vi "HFRR ADV v01.vi"() -> ()   [LabVIEW 2025] (continued)
        n1012 = property on="Analysis" class="Bool (strict)"("DisabledEnum"=w970) -> ()  [unwired: 2 in, 2 out]
        n1013 = property on="Home" class="Bool (strict)"("DisabledEnum"=w970) -> ()  [unwired: 2 in, 2 out]
        n1014 = property on="Report" class="Bool (strict)"("DisabledEnum"=w970) -> ()  [unwired: 2 in, 2 out]
        n1015 = property on="Main Dashboard Buttons" class="RadioBtnsControl (strict)"("DisabledEnum"=w970) -> ()  [unwired: 2 in, 2 out]
        n1016 = case shown="True" w969 {
          tunnel: [T15."Disabled" ("Disabled") T15."Enabled" ("Disabled")] -> w968
          frame False {
          }
          frame True {
          }
        }
        n1017 = property on="About" class="Bool (strict)"("DisabledEnum"=w968) -> ()  [unwired: 2 in, 2 out]
      }
      frame "Test Setup" {
        w975 = T15."Enabled" ("Disabled")
        n1018 = local read "Service Password enable"() -> (w974:bool)
        n1019 = property on="Dashboard" class="Bool (strict)"("DisabledEnum"=T15."Disabled" ("Disabled")) -> ()  [unwired: 2 in, 2 out]
        n1020 = property on="Imaging" class="Bool (strict)"("DisabledEnum"=w975) -> ()  [unwired: 2 in, 2 out]
        n1021 = property on="Analysis" class="Bool (strict)"("DisabledEnum"=w975) -> ()  [unwired: 2 in, 2 out]
        n1022 = property on="Home" class="Bool (strict)"("DisabledEnum"=w975) -> ()  [unwired: 2 in, 2 out]
        n1023 = property on="Report" class="Bool (strict)"("DisabledEnum"=w975) -> ()  [unwired: 2 in, 2 out]
        n1024 = property on="Test Setup" class="Bool (strict)"("DisabledEnum"=w975) -> ()  [unwired: 2 in, 2 out]
        n1025 = case shown="True" w974 {
          tunnel: [T15."Disabled" ("Disabled") T15."Enabled" ("Disabled")] -> w973
          frame False {
          }
          frame True {
          }
        }
        n1026 = property on="About" class="Bool (strict)"("DisabledEnum"=w973) -> ()  [unwired: 2 in, 2 out]
      }
      frame "Adv Scar" {
        w982 = T15."Enabled" ("Disabled")
        n1027 = property on="Dashboard" class="Bool (strict)"("DisabledEnum"=T15."Disabled" ("Disabled")) -> ()  [unwired: 2 in, 2 out]
        n1028 = property on="Imaging" class="Bool (strict)"("DisabledEnum"=w982) -> ()  [unwired: 2 in, 2 out]
        n1029 = property on="Analysis" class="Bool (strict)"("DisabledEnum"=w982) -> ()  [unwired: 2 in, 2 out]
        n1030 = property on="Home" class="Bool (strict)"("DisabledEnum"=w982) -> ()  [unwired: 2 in, 2 out]
        n1031 = property on="Report" class="Bool (strict)"("DisabledEnum"=w982) -> ()  [unwired: 2 in, 2 out]
        n1032 = property on="Test Setup" class="Bool (strict)"("DisabledEnum"=w982) -> ()  [unwired: 2 in, 2 out]
        n1033 = local read "Service Password enable"() -> (w980:bool)
        n1034 = case shown="True" w980 {
          tunnel: [T15."Disabled" ("Disabled") T15."Enabled" ("Disabled")] -> w979
          frame False {
          }
          frame True {
          }
        }
        n1035 = property on="About" class="Bool (strict)"("DisabledEnum"=w979) -> ()  [unwired: 2 in, 2 out]
      }
      frame "Adv Scar Report" {
        w987 = T15."Enabled" ("Disabled")
        n1036 = property on="Dashboard" class="Bool (strict)"("DisabledEnum"=T15."Disabled" ("Disabled")) -> ()  [unwired: 2 in, 2 out]
        n1037 = property on="Imaging" class="Bool (strict)"("DisabledEnum"=w987) -> ()  [unwired: 2 in, 2 out]
        n1038 = property on="Analysis" class="Bool (strict)"("DisabledEnum"=w987) -> ()  [unwired: 2 in, 2 out]
        n1039 = property on="Home" class="Bool (strict)"("DisabledEnum"=w987) -> ()  [unwired: 2 in, 2 out]
        n1040 = property on="Report" class="Bool (strict)"("DisabledEnum"=w987) -> ()  [unwired: 2 in, 2 out]
        n1041 = property on="Test Setup" class="Bool (strict)"("DisabledEnum"=w987) -> ()  [unwired: 2 in, 2 out]
        n1042 = local read "Service Password enable"() -> (w986:bool)
        n1043 = case shown="True" w986 {
          tunnel: [T15."Disabled" ("Disabled") T15."Enabled" ("Disabled")] -> w985
          frame False {
          }
          frame True {
          }
        }
        n1044 = property on="About" class="Bool (strict)"("DisabledEnum"=w985) -> ()  [unwired: 2 in, 2 out]
      }
      frame "Compare Files" {
        w993 = T15."Enabled" ("Disabled")
        n1045 = local read "Service Password enable"() -> (w992:bool)
        n1046 = property on="Dashboard" class="Bool (strict)"("DisabledEnum"=T15."Disabled" ("Disabled")) -> ()  [unwired: 2 in, 2 out]
        n1047 = property on="Imaging" class="Bool (strict)"("DisabledEnum"=w993) -> ()  [unwired: 2 in, 2 out]
        n1048 = property on="Analysis" class="Bool (strict)"("DisabledEnum"=w993) -> ()  [unwired: 2 in, 2 out]
        n1049 = property on="Home" class="Bool (strict)"("DisabledEnum"=w993) -> ()  [unwired: 2 in, 2 out]
        n1050 = property on="Report" class="Bool (strict)"("DisabledEnum"=w993) -> ()  [unwired: 2 in, 2 out]
        n1051 = property on="Test Setup" class="Bool (strict)"("DisabledEnum"=w993) -> ()  [unwired: 2 in, 2 out]
        n1052 = case shown="True" w992 {
          tunnel: [T15."Disabled" ("Disabled") T15."Enabled" ("Disabled")] -> w991
          frame False {
          }
          frame True {
          }
        }
        n1053 = property on="About" class="Bool (strict)"("DisabledEnum"=w991) -> ()  [unwired: 2 in, 2 out]
      }
      frame "Acquire" {
        n1054 = local read "Service Password enable"() -> (w997:bool)
        n1055 = property on="Test Setup" class="Bool (strict)"("DisabledEnum"=T15."Disabled" ("Disabled")) -> ()  [unwired: 2 in, 2 out]
        n1056 = local read "Auto Start Test"() -> (w999:bool)
        n1057 = local read "RUN"() -> (w1001:bool)
        n1058 = case shown="True" w997 {
          tunnel: [T15."Disabled" ("Disabled") T15."Enabled" ("Disabled")] -> w998
          frame False {
          }
          frame True {
          }
        }
        n1059 = Or(x=w1001, y=w999) -> (x .or. y?=w1000:bool)
        n1060 = case shown="True" w1000 {
          tunnel: [T15."Enabled" ("Disabled") T15."Disabled" ("Disabled")] -> w1003
          frame False {
          }
          frame True {
          }
        }
        n1061 = property on="About" class="Bool (strict)"("DisabledEnum"=w998) -> ()  [unwired: 2 in, 2 out]
        n1062 = property on="Imaging" class="Bool (strict)"("DisabledEnum"=w1003) -> ()  [unwired: 2 in, 2 out]
        n1063 = property on="Dashboard" class="Bool (strict)"("DisabledEnum"=w1003) -> ()  [unwired: 2 in, 2 out]
        n1064 = property on="Analysis" class="Bool (strict)"("DisabledEnum"=w1003) -> ()  [unwired: 2 in, 2 out]
        n1065 = property on="Home" class="Bool (strict)"("DisabledEnum"=w1003) -> ()  [unwired: 2 in, 2 out]
        n1066 = property on="Report" class="Bool (strict)"("DisabledEnum"=w1003) -> ()  [unwired: 2 in, 2 out]
      }
      frame "About" {
        n1067 = local read "FILE"() -> (w1016:string)
        n1068 = local read "TEST FILE NAM,E SAVED"() -> (w1009:bool)
        n1069 = call <vilib>:"Trim Whitespace.vi"("string"=w1016) -> ("trimmed string"=w1015:string)  [unwired: 1 in]
        n1070 = local read "Auto Start Test"() -> (w1019:bool)
        n1071 = String Length(string=w1015) -> (length=w1014:i32)
        n1072 = Greater?(x=w1014, y=1) -> (0:w1011:bool)
        n1073 = And(x=w1011, y=w1009) -> (x .and. y?=w1010:bool)
        n1074 = local read "RUN"() -> (w1021:bool)
        n1075 = case shown="True" w1010 {
          tunnel: [T15."Disabled" ("Disabled") T15."Enabled" ("Disabled")] -> w1012
          frame False {
          }
          frame True {
          }
        }
        n1076 = Or(x=w1021, y=w1019) -> (x .or. y?=w1020:bool)
        n1077 = property on="About" class="Bool (strict)"("DisabledEnum"=T15."Enabled" ("Disabled")) -> ()  [unwired: 2 in, 2 out]
        n1078 = case shown="False" w1020 {
          tunnel: [T15."Enabled" ("Disabled") T15."Disabled" ("Disabled")] -> w1018
          frame False {
          }
          frame True {
          }
        }
        n1079 = property on="Dashboard" class="Bool (strict)"("DisabledEnum"=w1012) -> ()  [unwired: 2 in, 2 out]
        n1080 = property on="Test Setup" class="Bool (strict)"("DisabledEnum"=T15."Disabled" ("Disabled")) -> ()  [unwired: 2 in, 2 out]
        n1081 = property on="Imaging" class="Bool (strict)"("DisabledEnum"=w1018) -> ()  [unwired: 2 in, 2 out]
        n1082 = property on="Analysis" class="Bool (strict)"("DisabledEnum"=w1018) -> ()  [unwired: 2 in, 2 out]
        n1083 = property on="Home" class="Bool (strict)"("DisabledEnum"=w1018) -> ()  [unwired: 2 in, 2 out]
        n1084 = property on="Report" class="Bool (strict)"("DisabledEnum"=w1018) -> ()  [unwired: 2 in, 2 out]
      }
    }
    n1085 = local read "Quit"() -> (w952:bool)
    "Single" <- "Single - Graph"
  }
  n1086 = disable-structure shown="Disabled" {
    disable-tunnel: [w1289 _] -> w36
    disable-tunnel: _ -> [w1288 _]
    frame Disabled {
      n1087 = while {
        tunnel: w1288 -> [_]
        tunnel: [w1290] -> w1289
        tunnel: [w1291] -> _
        i -> [w1291]
        stop <- w1290 stop-if-true
        w1307 = u16 10 items=["1.0"=10, "1.5"=15, "2.0"=20] ("stop bits (10: 1 bit)")
        n1088 = Wait (ms)(milliseconds to wait=u32 10) -> ()  [unwired: 1 out]
        n1089 = call-poly "VISA Configure Serial Port"("VISA resource name"=refnum<visa-resource-name> "ASRL1::INSTR" ("COM PORT"), "timeout (10sec)"=u32 10, "baud rate (9600)"=u32 57600, "data bits (8)"=u16 8, "stop bits (10: 1 bit)"=w1307) -> ("VISA resource name out"=w1293:refnum<visa-resource-name>, "error out"=w1302:errorcluster)  [unwired: 9 in]
        n1090 = VISA Read(VISA resource name=w1293, byte count=u32 2 ("byte count (0)")) -> (read buffer=w1301:string)  [unwired: 1 in, 3 out]
        n1091 = String Subset(string=w1301, offset (0)=0, length (rest)=2 ("length (rest)")) -> (substring=w1300:string)
        n1092 = Match Pattern(string=w1300, regular expression="<>") -> (offset past match=w1297:i32)  [unwired: 1 in, 3 out]
        n1093 = Greater Or Equal?(x=w1297, y=0) -> (x >= y?=w1292:bool)
        n1094 = case shown="True" w1292 {
          tunnel: w1293 -> [_ w1311]
          tunnel: w1302 -> [_ w1310]
          frame False {
          }
          frame True {
            n1095 = VISA Read(VISA resource name=w1311, byte count=u32 32 ("byte count (0)"), error in (no error)=w1310) -> (read buffer=w1309:string)  [unwired: 3 out]
            n1096 = String Subset(string=w1309, offset (0)=0, length (rest)=8 ("length (rest)")) -> (substring=w1313:string)
            n1097 = String Subset(string=w1309, offset (0)=8, length (rest)=8 ("length (rest)")) -> (substring=w1314:string)
            n1098 = Decimal String To Number(string=w1314) -> (number=w1321:i32)  [unwired: 2 in, 1 out]
            n1099 = Decimal String To Number(string=w1313) -> (number=w1317:i32)  [unwired: 2 in, 1 out]
            n1100 = Divide(x=w1321, y=10000) -> ()  [unwired: 1 out]
            n1101 = Divide(x=w1317, y=1000000) -> ()  [unwired: 1 out]
          }
        }
        n1102 = local read "Quit"() -> (w1290:bool)
      }
    }
    frame Enabled {
    }
  }
  n1103 = local write "Err Count"(0 ("Err Count")) -> ()
  n1104 = local write "FRICVALZ"(0.0 ("FRICVALZ")) -> ()
  n1105 = while {
    shift-right: [w1337] -> w50
    shift-left: _ -> [w1328]
    shift-right: [w1336] -> w49
    shift-left: errorcluster {"status"=TRUE, "code"=0, "source"="Init"} ("error IO") -> [w1330]
    tunnel: [w1324] -> w39
    tunnel: [w1335] -> _
    i -> [w1335]
    stop <- w1324 stop-if-true
    n1106 = local read "Port 1a"() -> (w1331:bool)
    n1107 = local read "Port 3"() -> (w1332:bool)
    n1108 = local read "Com Port 1"() -> (w1329:refnum<visa-resource-name>)
    n1109 = Or(x=w1332, y=w1331) -> (x .or. y?=w1334:bool)
    n1110 = Unbundle(w1330) -> ("status"=→"Port 3":bool)  [unwired: 2 out]
    n1111 = Not Equal?(x=w1329, y=w1328) -> (x != y?=w1327:bool)
    n1112 = case shown="True" w1334 {
      frame False {
        w1340 = FALSE ("Visible")
        n1113 = property on="Port 1a" class="Bool (strict)"("Visible"=w1340) -> ()  [unwired: 2 in, 2 out]
        n1114 = property on="Port 3" class="Bool (strict)"("Visible"=w1340) -> ()  [unwired: 2 in, 2 out]
      }
      frame True {
        w1341 = TRUE ("Visible")
        n1115 = property on="Port 1a" class="Bool (strict)"("Visible"=w1341) -> ()  [unwired: 2 in, 2 out]
        n1116 = property on="Port 3" class="Bool (strict)"("Visible"=w1341) -> ()  [unwired: 2 in, 2 out]
      }
    }
    n1117 = Or(x=w1327, y="Re-initialize Port1") -> (x .or. y?=w1325:bool)
    n1118 = case shown="True" w1325 {
      tunnel: [w1338 errorcluster {"status"=TRUE, "code"=0, "source"="Init"} ("error out")] -> w1326
      tunnel: w1330 -> [w1338 _]
      frame False {
      }
      frame True {
      }
    }
    n1119 = case shown="Error" w1326 {
      selector: w1326 -> [w1348 w1375]
      tunnel: [w1351 w1379] -> w1337
      tunnel: [w1350 w1373] -> w1336
      tunnel: w1328 -> [w1349 w1377]
      frame No Error {
        n1120 = property class="Instr"(reference=w1349, error in=w1348) -> (reference out=w1346:refnum<visa-resource-name>, error out=w1347:errorcluster, "Serial Settings:Number of Bytes at Serial Port"=w1342:u32)
        "Port 1" <- w1342
        n1121 = Greater?(x=w1342, y=u32 5) -> (0:w1344:bool)
        n1122 = Not(x=w1344) -> (.not. x?=→"Port 1a":bool)
        n1123 = while {
          tunnel: [w1368] -> w1350
          tunnel: [w1367] -> w1351
          tunnel: w1347 -> [w1366]
          tunnel: w1346 -> [w1365]
          stop <- TRUE stop-if-true
          n1124 = property class="Instr" props=["Serial Settings:Number of Bytes at Serial Port"](reference=w1365, error in=w1366) -> (reference out=w1370:refnum<visa-resource-name>, error out=w1369:errorcluster)  [unwired: 1 out]
          n1125 = VISA Read(VISA resource name=w1370, byte count=u32 1000, error in (no error)=w1369) -> (VISA resource name out=w1367:refnum<visa-resource-name>, read buffer=w1352:string, error out=w1368:errorcluster)  [unwired: 1 out]
          "UnoRead" <- w1352
          n1126 = Spreadsheet String To Array(delimiter (Tab)=";", format string="", spreadsheet string=w1352, array type (2D Dbl)=dbl[] []) -> (array=w1362:dbl[])
          n1127 = Index Array(array=w1362) -> (element #1=→"LVDT MIN":dbl, element #2=→"LVDT MAX":dbl, element #3=→"LVDT Peak":dbl, element #4=→"pizo raw":dbl, element #5=→"Friction":dbl, element #6=→"cof 2":dbl)  [unwired: 6 in]
        }
      }
      frame Error {
        w1385 = u16 0 items=["None", "XON/XOFF", "RTS/CTS", "XON/XOFF & RTS/CTS", "DTR/DSR", "XON/XOFF & DTR/DSR"] ("flow control (0:none)  2")
        w1383 = u16 10 items=["1.0"=10, "1.5"=15, "2.0"=20] ("stop bits 2")
        w1381 = u16 0 items=["None", "Odd", "Even", "Mark", "Space"] ("parity 2")
        w1382 = u32 10000  # timeout (10sec)
        n1128 = VISA Close(VISA resource name=w1377, error in (no error)=w1375) -> (error out=w1378:errorcluster)
        n1129 = local write "Port 1a"(FALSE ("Port 1a")) -> ()
        n1130 = local read "Com Port 1"() -> (w1372:refnum<visa-resource-name>)
        n1131 = call <vilib>:"Clear Errors.vi"("error in (no error)"=w1378) -> ("error out"=w1376:errorcluster)  [unwired: 5 in, 1 out]
        n1132 = call-poly "VISA Configure Serial Port"("VISA resource name"=w1372, "timeout (10sec)"=w1382, "baud rate (9600)"=u32 250000 ("baud rate  2"), "data bits (8)"=u16 8 ("data bits  2"), "parity (0:none)"=w1381, "error in (no error)"=w1376, "stop bits (10: 1 bit)"=w1383, "flow control (0:none)"=w1385) -> ("VISA resource name out"=w1386:refnum<visa-resource-name>, "error out"=w1387:errorcluster)  [unwired: 6 in]
        n1133 = flat-sequence {
          tunnel: w1386 -> [w1389]
          tunnel: w1387 -> [w1388]
          tunnel: [w1389] -> w1379
          tunnel: [w1388] -> w1373
          frame #0 {
            n1134 = Wait (ms)(milliseconds to wait=u32 50) -> ()  [unwired: 1 out]
          }
        }
        "Residual Uno" <- ""
        "Port 1 Error" <- w1373
      }
    }
    n1135 = local read "Quit"() -> (w1324:bool)
    "Error Uno" <- w1330
  }
  n1136 = while {
    shift-right: [w1406] -> w34
    shift-left: _ -> [w1397]
    shift-right: [w1405] -> w33
    shift-left: errorcluster {"status"=FALSE, "code"=0, "source"="Init"} ("error out") -> [w1399]
    tunnel: [w1393] -> w38
    tunnel: [w1404] -> _
    i -> [w1404]
    stop <- w1393 stop-if-true
    n1137 = local read "Com Port 2"() -> (w1398:refnum<visa-resource-name>)
    n1138 = local read "Port 2a"() -> (w1400:bool)
    n1139 = Unbundle(w1399) -> ("status"=→"Port 4":bool)  [unwired: 2 out]
    n1140 = call <vilib>:"High Resolution Polling Wait.vi"("seconds to wait"=0.2) -> ()  [unwired: 10 in, 1 out]
    n1141 = local read "Port 4"() -> (w1401:bool)
    n1142 = Not Equal?(x=w1398, y=w1397) -> (x != y?=w1396:bool)
    n1143 = Or(x=w1401, y=w1400) -> (x .or. y?=w1403:bool)
    n1144 = Or(x=w1396, y="Re-initialize Port2") -> (x .or. y?=w1394:bool)
    n1145 = case shown="True" w1403 {
      frame False {
        w1409 = FALSE ("Visible")
        n1146 = property on="Port 2a" class="Bool (strict)"("Visible"=w1409) -> ()  [unwired: 2 in, 2 out]
        n1147 = property on="Port 4" class="Bool (strict)"("Visible"=w1409) -> ()  [unwired: 2 in, 2 out]
      }
      frame True {
        w1410 = TRUE ("Visible")
        n1148 = property on="Port 2a" class="Bool (strict)"("Visible"=w1410) -> ()  [unwired: 2 in, 2 out]
        n1149 = property on="Port 4" class="Bool (strict)"("Visible"=w1410) -> ()  [unwired: 2 in, 2 out]
      }
    }
    n1150 = case shown="True" w1394 {
      tunnel: [w1407 errorcluster {"status"=TRUE, "code"=0, "source"="Init"} ("error out")] -> w1395
      tunnel: w1399 -> [w1407 _]
      frame False {
      }
      frame True {
      }
    }
    n1151 = case shown="No Error" w1395 {
      selector: w1395 -> [w1432 w1462]
      tunnel: [w1412 w1467] -> w1406
      tunnel: [w1433 w1460] -> w1405
      tunnel: w1397 -> [w1436 w1465]
      tunnel: [w1435 _] -> _
      frame No Error {
        n1152 = property class="Instr"(reference=w1436, error in=w1432) -> (reference out=w1419:refnum<visa-resource-name>, error out=w1431:errorcluster, "Serial Settings:Number of Bytes at Serial Port"=w1415:u32)
        "Port 2" <- w1415
        n1153 = while {
          tunnel: [w1443] -> w1427
          tunnel: [w1442] -> w1428
          tunnel: w1431 -> [w1441]
          tunnel: w1419 -> [w1440]
          tunnel: [w1439] -> _
          i -> [w1439]
          stop <- TRUE stop-if-true
          n1154 = property class="Instr" props=["Serial Settings:Number of Bytes at Serial Port"](reference=w1440, error in=w1441) -> (reference out=w1445:refnum<visa-resource-name>, error out=w1444:errorcluster)  [unwired: 1 out]
          n1155 = VISA Read(VISA resource name=w1445, byte count=u32 1000, error in (no error)=w1444) -> (VISA resource name out=w1442:refnum<visa-resource-name>, error out=w1443:errorcluster)  [unwired: 2 out]
        }
        n1156 = Greater?(x=w1415, y=u32 23) -> (0:w1417:bool)
        n1157 = Not(x=w1417) -> ()  [unwired: 1 out]
        n1158 = local read "Due Com"() -> (w1420:string[])
        n1159 = call "Elapsed Time10"("Time Target (s)"=2.0, "Reset"=w1417, "Auto Reset"=FALSE) -> ("Time has Elapsed"=→"Port 2a":bool)  [unwired: 9 in, 7 out]
        n1160 = Array Size(array=w1420) -> (size(s)=w1435:i32)
        n1161 = Delete From Array(array=w1420, length=1, index=0) -> (deleted portion=w1423:string[], array with subset deleted=w1424:string[])
        n1162 = local write "Due Com"(w1424) -> ()
        n1163 = Index Array(array=w1423, index=0) -> (element=w1421:string)
        n1164 = Not Equal?(x=w1421, y="") -> (x != y?=w1429:bool)
        n1165 = case shown="True" w1429 {
          tunnel: w1428 -> [w1447 w1452]
          tunnel: [w1447 w1456] -> w1434
          tunnel: w1427 -> [w1446 w1451]
          tunnel: [w1446 w1454] -> w1433
          tunnel: w1421 -> [_ w1450]
          tunnel: [_ w1453] -> _
          frame False {
            # "DATA  WRITE LOOP"
          }
          frame True {
            n1166 = Concatenate Strings(w1450, "\r\n") -> (w1449:string)
            n1167 = VISA Write(VISA resource name=w1452, write buffer=w1449, error in (no error)=w1451) -> (VISA resource name out=w1456:refnum<visa-resource-name>, return count=w1453:u32, error out=w1455:errorcluster)
            n1168 = flat-sequence {
              tunnel: w1455 -> [w1457]
              tunnel: [w1457] -> w1454
              frame #0 {
                n1169 = Wait (ms)(milliseconds to wait=u32 5) -> ()  [unwired: 1 out]
              }
            }
          }
        }
        n1170 = VISA Flush I/O Buffer(VISA resource name=w1434) -> (VISA resource name out=w1412:refnum<visa-resource-name>, error out=→"error out 9":errorcluster)  [unwired: 2 in]
      }
      frame Error {
        w1473 = u16 0 items=["None", "XON/XOFF", "RTS/CTS", "XON/XOFF & RTS/CTS", "DTR/DSR", "XON/XOFF & DTR/DSR"] ("flow control (0:none)  2")
        w1471 = u16 10 items=["1.0"=10, "1.5"=15, "2.0"=20] ("stop bits 2")
        w1469 = u16 0 items=["None", "Odd", "Even", "Mark", "Space"] ("parity 2")
        w1470 = u32 10000  # timeout (10sec)
        n1171 = VISA Clear(VISA resource name=w1465, error in (no error)=w1462) -> (VISA resource name out=w1464:refnum<visa-resource-name>, error out=w1463:errorcluster)
        n1172 = VISA Close(VISA resource name=w1464, error in (no error)=w1463) -> (error out=w1466:errorcluster)
        n1173 = call <vilib>:"Clear Errors.vi"("error in (no error)"=w1466) -> ()  [unwired: 5 in, 2 out]
        n1174 = local read "Com Port 2"() -> (w1459:refnum<visa-resource-name>)
        "visa due" <- w1459
        n1175 = call-poly "VISA Configure Serial Port"("VISA resource name"=w1459, "timeout (10sec)"=w1470, "baud rate (9600)"=u32 250000 ("baud rate  2"), "data bits (8)"=u16 8 ("data bits  2"), "parity (0:none)"=w1469, "stop bits (10: 1 bit)"=w1471, "flow control (0:none)"=w1473) -> ("VISA resource name out"=w1474:refnum<visa-resource-name>, "error out"=w1475:errorcluster)  [unwired: 7 in]
        n1176 = flat-sequence {
          tunnel: w1474 -> [w1477]
          tunnel: w1475 -> [w1476]
          tunnel: [w1477] -> w1467
          tunnel: [w1476] -> w1460
          frame #0 {
            n1177 = Wait (ms)(milliseconds to wait=u32 50) -> ()  [unwired: 1 out]
          }
        }
        "Residual Due" <- ""
        "Port 2 Error" <- w1460
      }
    }
    n1178 = local read "Quit"() -> (w1393:bool)
    "Error Due" <- w1399
  }
  n1179 = property on="RUN" class="Bool (strict)"("Visible"=TRUE) -> ()  [unwired: 2 in, 2 out]
  n1180 = while {
    tunnel: [w1495] -> _
    tunnel: [w1479] -> w52
    i -> [w1495]
    stop <- w1479 stop-if-true
    n1181 = local read "conststatus"() -> (w1483:dbl)
    n1182 = local read "Main Tab"() -> (w1481:T2)
    n1183 = local read "EDIT"() -> (w1501:bool)
    n1184 = local read "Rate"() -> (w1500:dbl)
    n1185 = case shown="True" w1501 {
      tunnel: [FALSE TRUE] -> w1487
      frame False {
      }
      frame True {
      }
    }
    n1186 = property on="Time slide" class="Slide (strict)"("Scale.Range:Maximum"=2500.0) -> ()  [unwired: 2 in, 2 out]
    n1187 = Equal?(x=w1481, y=T22."About" ("Main Tab")) -> (x = y?=w1493:bool)
    n1188 = Equal?(x=w1483, y=0.0) -> (x = y?=w1484:bool)
    n1189 = Divide(x=1.0, y=w1500) -> (x/y=w1496:dbl)
    "Time 2" <- w1496
    n1190 = case shown="True" w1484 {
      frame False {
      }
      frame True {
        # "C:\\WinDucom\\calibrate WO 2391.dcf"
        n1191 = local write "Lan flag"(22) -> ()
        n1192 = local write "conststatus"(10.0 ("rpm value : 2")) -> ()
        n1193 = String To Path(string="C:\\LAB-IQ\\calibrate WO 2465.dcf") -> (path=w1507:path)
        n1194 = Open/Create/Replace File "Open File"(file path (use dialog)=w1507) -> (refnum out=w1505:refnum<file>)  [unwired: 5 in, 2 out]
        n1195 = for {
          N: 23 -> [_]
          tunnel: w1505 -> [w1516]
          i -> [w1510]
          (unwired) TRUE ("line mode (F)")
          n1196 = Read from Text File "Read File"(file (use dialog)=w1516) -> (text=w1515:string)  [unwired: 3 in, 3 out]
          n1197 = Match Pattern(string=w1515, regular expression="]") -> (after substring=w1513:string)  [unwired: 1 in, 3 out]
          n1198 = String Subset(string=w1515, offset (0)=5, length (rest)=10 ("length (rest)")) -> (substring=w1508:string)
          n1199 = Fract/Exp String To Number(string=w1508) -> (number=w1509:dbl)  [unwired: 3 in, 1 out]
          n1200 = Match Pattern(string=w1513, regular expression="-") -> (before substring=w1511:string)  [unwired: 1 in, 3 out]
          n1201 = case shown="16" w1510 {
            tunnel: w1509 -> [w1519 w1520 w1521 w1522 _ _ _ w1527 w1528 _ w1529 w1530 w1531 w1532 w1533 w1534 _ w1535 w1536 _ _ _ _ _]
            tunnel: w1511 -> [_ _ _ _ w1523 w1524 w1525 _ _ _ _ _ _ _ _ _ _ _ _ w1537 w1538 _ w1539 _]
            frame 0 {
              n1202 = local write "FRIC. FORCE :"(w1519) -> ()
            }
            frame 1 {
              n1203 = local write "TEMPERATURE :"(w1520) -> ()
            }
            frame 2 {
              n1204 = local write "HUMIDITY:"(w1521) -> ()
            }
            frame 3 {
              n1205 = local write "AIR TEMPERATURE :"(w1522) -> ()
            }
            frame 4 {
              n1206 = local write "Com Port 1"(w1523) -> ()
            }
            frame 5 {
              n1207 = local write "Com Port 2"(w1524) -> ()
              n1208 = local write "visa due"(w1524) -> ()
            }
            frame 6 {
              n1209 = String To Path(string=w1525) -> (path=w1526:path)
              n1210 = local write "File Path"(w1526) -> ()
              "String" <- w1525
            }
            frame 7 {
              n1211 = local write "DISPLACEMENT :"(w1527) -> ()
            }
            frame 8 {
              n1212 = local write "STROKE GAIN :"(w1528) -> ()
            }
            frame 9 {
            }
            frame 10 {
              n1213 = local write "Language Selection"(w1529) -> ()
            }
            frame 11 {
              n1214 = local write "CH-POWER +"(w1530) -> ()
            }
            frame 12 {
              n1215 = local write "CH-POWER -"(w1531) -> ()
            }
            frame 13 {
              n1216 = local write "CH-HEATER"(w1532) -> ()
            }
            frame 14 {
              n1217 = local write "CH-HUMIDITY WET"(w1533) -> ()
            }
            frame 15 {
              n1218 = local write "CH-HUMIDITY DRY"(w1534) -> ()
            }
            frame 16 {
            }
            frame 17 {
              n1219 = local write "AIR TEMP INTERCEPT:"(w1535) -> ()
            }
            frame 18 {
              n1220 = local write "TEMP INTERCEPT:"(w1536) -> ()
            }
            frame 19 {
              n1221 = local write "S.NO"(w1537) -> ()
            }
            frame 20 {
              n1222 = local write "Com Port 3"(w1538) -> ()
            }
            frame 21 {
            }
            frame 22 {
              n1223 = local write "C3 :"(w1539) -> ()
            }
            frame 23, Default {
            }
          }
        }
      }
    }
    n1224 = Select(t=u32 2500 ("milliseconds to wait"), s=w1493, f=u32 500 ("milliseconds to wait")) -> (s? t:f=w1491:u32)
    n1225 = Multiply(x=w1496, y=w1491) -> (x*y=w1498:dbl)
    n1226 = property on="FF Calibration g" class="WFGraph (strict)"("Visible"=w1487) -> ()  [unwired: 2 in, 2 out]
    n1227 = property on="Lift" class="Bool (strict)"("Visible"=w1487) -> ()  [unwired: 2 in, 2 out]
    n1228 = property on="Time slide" class="Slide (strict)"("Visible"=w1487) -> ()  [unwired: 2 in, 2 out]
    n1229 = call "Elapsed Time2"("Time Target (s)"=w1498, "Auto Reset"=TRUE) -> ("Time has Elapsed"=w1488:bool)  [unwired: 10 in, 7 out]
    n1230 = case shown="True" w1488 {
      frame False {
        # "79.77669138"
        # "2.3554"
        "Err Count" <- 0 ("y")
      }
      frame True {
        n1231 = stacked-sequence {
          frame #0 {
            n1232 = stacked-sequence {
              frame #0 {
                "Lift" <- TRUE ("Lift")
              }
            }
          }
          frame #1 {
          }
          frame #2 {
          }
          frame #3 {
            w1542 = 0.0
            # "DATA PROCESSING"
            # "115 mV/N"
            n1233 = local read "RH Numeric:"() -> (w1548:dbl)
            n1234 = local read "HUMIDITY:"() -> (w1549:dbl)
            n1235 = Multiply(x=w1548, y=w1549) -> (x*y=→"Humidity ( %RH )" →"Hum" →"Hum 2":dbl)
            n1236 = local read "Friction"() -> (w1543:dbl)
            n1237 = local write "TEMP"(w1542) -> ()
            n1238 = local read "FRICVALZ"() -> (w1560:dbl)
            n1239 = Compound Arithmetic op=OR("FRICVALZ 4", "FRICVALZ 3", "FRICVALZ 2") -> (w1551:bool)
            n1240 = case shown="True" w1551 {
              tunnel: w1543 -> [_ w1566]
              frame False {
              }
              frame True {
                w1565 = FALSE ("FRICVALZ")
                n1241 = local write "FRICVALZ 3"(w1565) -> ()
                n1242 = local write "FRICVALZ 2"(w1565) -> ()
                n1243 = local write "FRICVALZ 4"(w1565) -> ()
                "FRICVALZ" <- w1566
              }
            }
            n1244 = Subtract(x=w1543, y=w1560) -> (x-y=w1555:dbl)
            "FF 2" <- w1555
            "FF 4" <- w1555
            n1245 = local write "FF 3"(w1555) -> ()
            n1246 = local read "TEMP"() -> (w1559:dbl)
            n1247 = Not A Number/Path/Refnum?(number/path/refnum=w1555) -> (NaN/Path/Refnum?=w1557:bool)
            n1248 = Divide(x=w1555, y=1.96) -> (x/y=w1552:dbl)
            n1249 = Not A Number/Path/Refnum?(number/path/refnum=w1559) -> (NaN/Path/Refnum?=w1558:bool)
            n1250 = Compound Arithmetic op=OR(w1558, w1557) -> (w1556:bool)
            n1251 = Not A Number/Path/Refnum?(number/path/refnum=w1552) -> (NaN/Path/Refnum?=w1553:bool)
            n1252 = case shown="True" w1556 {
              frame False {
              }
              frame True {
                n1253 = local write "TEMP"(0.0 ("TEMP")) -> ()
                n1254 = local write "FF 2"(0.0 ("FF 2")) -> ()
                n1255 = local write "reinit"(TRUE ("reinit")) -> ()
              }
            }
            n1256 = Select(t=0.0, s=w1553, f=w1552) -> (s? t:f=→"COF 2":dbl)
            "AIR TEMP" <- w1542
            "TEMP 2" <- w1542
            "TEMP 3" <- w1542
          }
          frame #4 {
          }
        }
      }
    }
    n1257 = Wait (ms)(milliseconds to wait=u32 50) -> ()  [unwired: 1 out]
    n1258 = local read "Quit"() -> (w1479:bool)
    "Rate" <- 2500.0 ("No of Samples")
    "Humid Last buf" <- dbl[] [0.0, 0.0, 0.0, 0.0] ("Humid Last buf")
  }
  n1259 = while {
    tunnel: w55 -> [_]
    tunnel: [w1594] -> _
    tunnel: [w1569] -> w54
    i -> [w1594]
    stop <- w1569 stop-if-true
    # "C:\\LAB-IQ-NXT\\Scar View.exe"
    n1260 = local read "OK Button 16"() -> (w1583:bool)
    n1261 = local read "Re-Initialise"() -> (w1579:bool)
    n1262 = local read "Main Tab"() -> (w1575:T2)
    n1263 = local read "service 3"() -> (w1576:bool)
    n1264 = local read "OPEN 6"() -> (w1578:bool)
    n1265 = local read "EDIT 2"() -> (w1581:bool)
    n1266 = flat-sequence {
      frame #0 {
        n1267 = local read "SAVE 2"() -> (w2197:bool)
        n1268 = stacked-sequence {
          frame #0 {
            n1269 = local read "EDIT"() -> (w2251:bool)
            n1270 = case shown="True" w2251 {
              tunnel: [u8 2 ("Disabled") u8 0 ("Disabled")] -> _
              frame False {
                w2253 = FALSE
                n1271 = local write "Password"("") -> ()
                n1272 = property on="SrvM CP" class="Bool (strict)"("Visible"=w2253) -> ()  [unwired: 2 in, 2 out]
                n1273 = property on="message" class="Str"("Visible"=w2253) -> ()  [unwired: 2 in, 2 out]
                n1274 = local write "x = y?"(w2253) -> ()
                n1275 = property on="Password" class="Str"("Visible"=w2253) -> ()  [unwired: 2 in, 2 out]
                n1276 = property on="ENTER THE NEW PASSWORD" class="Str"("Visible"=w2253) -> ()  [unwired: 2 in, 2 out]
                n1277 = property on="ENTER CURRENT PASSWORD" class="Str"("Visible"=w2253) -> ()  [unwired: 2 in, 2 out]
                n1278 = local write "SrvM CP"(w2253) -> ()
              }
              frame True {
                w2256 = TRUE
                n1279 = property on="SrvM CP" class="Bool (strict)"("Visible"=w2256) -> ()  [unwired: 2 in, 2 out]
                n1280 = property on="Password" class="Str"("Visible"=w2256) -> ()  [unwired: 2 in, 2 out]
              }
            }
            "dipl pwd" <- "@143$\n" ("dipl pwd")
          }
          frame #1 {
            # "Gain password"
            n1281 = String To Byte Array(string="ENTER CURRENT PASSWORD") -> (unsigned byte array=w2261:u8[])
            n1282 = Search 1D Array(1D array=w2261, element=u8 10) -> (index of element=w2264:i32)  [unwired: 1 in]
            n1283 = Index Array(array=w2261, index=w2264) -> (element=w2260:u8)
            n1284 = Equal?(x=w2260, y=10) -> (x = y?=w2258:bool)
            n1285 = case shown="True" w2258 {
              frame False {
                n1286 = property on="ENTER THE NEW PASSWORD" class="Str"("Visible"=FALSE) -> ()  [unwired: 2 in, 2 out]
              }
              frame True {
                # "password"
                # "change password logic"
                n1287 = local read "ENTER CURRENT PASSWORD"() -> (w2277:string)
                n1288 = local read "dipl pwd"() -> (w2271:string)
                n1289 = String To Byte Array(string=w2277) -> (unsigned byte array=w2279:u8[])
                n1290 = String To Byte Array(string=w2271) -> (unsigned byte array=w2272:u8[])
                n1291 = Array Size(array=w2279) -> (size(s)=w2276:i32)
                n1292 = Array Size(array=w2272) -> (size(s)=w2274:i32)
                n1293 = for {
                  N: w2276 -> [_]
                  tunnel: w2279 -> [w2303]
                  tunnel: [w2301] -> w2280 mode=indexing
                  tunnel: w2276 -> [w2295]
                  i -> [w2296]
                  n1294 = Decrement(x=w2295) -> (x-1=w2293:i32)
                  n1295 = Equal?(x=w2296, y=w2293) -> (x = y?=w2294:bool)
                  n1296 = Index Array(array=w2303, index=w2296) -> (element=w2297:u8)
                  n1297 = Number To Decimal String(number=w2297) -> (decimal integer string=w2302:string)  [unwired: 1 in]
                  n1298 = Select(t="", s=w2294, f="\r") -> (s? t:f=w2299:string)
                  n1299 = Concatenate Strings(w2302, w2299) -> (w2301:string)
                }
                n1300 = for {
                  N: w2274 -> [_]
                  tunnel: w2272 -> [w2291]
                  tunnel: [w2289] -> w2273 mode=indexing
                  tunnel: w2274 -> [w2286]
                  i -> [w2287]
                  n1301 = Decrement(x=w2286) -> (x-1=w2285:i32)
                  n1302 = Equal?(x=w2287, y=w2285) -> (x = y?=w2284:bool)
                  n1303 = Index Array(array=w2291, index=w2287) -> (element=w2290:u8)
                  n1304 = Number To Decimal String(number=w2290) -> (decimal integer string=w2288:string)  [unwired: 1 in]
                  n1305 = Select(t="", s=w2284, f="\r") -> (s? t:f=w2281:string)
                  n1306 = Concatenate Strings(w2288, w2281) -> (w2289:string)
                }
                n1307 = local read "string"() -> (w2278:string)
                n1308 = Concatenate Strings(w2273) -> (w2267:string)
                n1309 = Concatenate Strings(w2278) -> (w2275:string)
                n1310 = Concatenate Strings(w2280) -> (w2268:string)
                n1311 = Equal?(x=w2268, y=w2275) -> (x = y?=w2270:bool)
                n1312 = Equal?(x=w2268, y=w2267) -> (x = y?=w2266:bool)
                n1313 = Or(x=w2270, y=w2266) -> (x .or. y?=w2269:bool)
                n1314 = case shown="True" w2269 {
                  frame False {
                  }
                  frame True {
                    n1315 = property on="ENTER THE NEW PASSWORD" class="Str"("Visible"=TRUE) -> ()  [unwired: 2 in, 2 out]
                  }
                }
              }
            }
          }
          frame #2 {
            n1316 = String To Byte Array(string="ENTER THE NEW PASSWORD") -> (unsigned byte array=w2306:u8[])
            n1317 = Search 1D Array(1D array=w2306, element=u8 10) -> (index of element=w2310:i32)  [unwired: 1 in]
            n1318 = Index Array(array=w2306, index=w2310) -> (element=w2308:u8)
            n1319 = Equal?(x=w2308, y=10) -> (x = y?=w2305:bool)
            n1320 = case shown="False" w2305 {
              frame False {
              }
              frame True {
                n1321 = local write "EDIT"(FALSE) -> ()
                n1322 = local write "SrvM CP"(FALSE) -> ()
                n1323 = local read "ENTER THE NEW PASSWORD"() -> (w2313:string)
                n1324 = String To Byte Array(string=w2313) -> (unsigned byte array=w2318:u8[])
                n1325 = Array Size(array=w2318) -> (size(s)=w2315:i32)
                n1326 = for {
                  N: w2315 -> [_]
                  tunnel: w2318 -> [w2331]
                  tunnel: [w2328] -> w2320 mode=indexing
                  tunnel: w2315 -> [w2323]
                  i -> [w2321]
                  n1327 = Decrement(x=w2323) -> (x-1=w2324:i32)
                  n1328 = Equal?(x=w2321, y=w2324) -> (x = y?=w2325:bool)
                  n1329 = Index Array(array=w2331, index=w2321) -> (element=w2330:u8)
                  n1330 = Number To Decimal String(number=w2330) -> (decimal integer string=w2329:string)  [unwired: 1 in]
                  n1331 = Select(t="", s=w2325, f="\r") -> (s? t:f=w2322:string)
                  n1332 = Concatenate Strings(w2329, w2322) -> (w2328:string)
                }
                n1333 = local read "file path"() -> (w2312:path)
                n1334 = Concatenate Strings(w2320) -> (w2314:string)
                n1335 = Delete(path (use dialog)=w2312) -> (deleted path=w2316:path)  [unwired: 4 in, 2 out]
                n1336 = call <vilib>:"Write Characters To File.vi"("append to file? (new file:F)"=FALSE, "character string"=w2314, "file path (dialog if empty)"=w2316) -> ()  [unwired: 2 in, 1 out]
              }
            }
          }
          frame #3 {
            n1337 = case shown="True" "SrvM CP" {
              frame False {
                w2334 = ""
                n1338 = local write "ENTER CURRENT PASSWORD"(w2334) -> ()
                n1339 = local write "ENTER THE NEW PASSWORD"(w2334) -> ()
                n1340 = property on="ENTER CURRENT PASSWORD" class="Str"("Visible"=FALSE) -> ()  [unwired: 2 in, 2 out]
              }
              frame True {
                n1341 = property on="ENTER THE NEW PASSWORD" class="Str"() -> ("Visible"=w2335:bool)  [unwired: 2 in, 2 out]
                n1342 = Not(x=w2335) -> (.not. x?=w2336:bool)
                n1343 = property on="ENTER CURRENT PASSWORD" class="Str"("Visible"=w2336) -> ()  [unwired: 2 in, 2 out]
              }
            }
          }
          frame #4 {
            n1344 = String To Byte Array(string="Password") -> (unsigned byte array=w2343:u8[])
            n1345 = Search 1D Array(1D array=w2343, element=u8 10) -> (index of element=w2341:i32)  [unwired: 1 in]
            n1346 = Index Array(array=w2343, index=w2341) -> (element=w2342:u8)
            n1347 = Equal?(x=w2342, y=10) -> (x = y?=w2338:bool)
            n1348 = case shown="True" w2338 {
              frame False {
              }
              frame True {
                # "password"
                # "password"
                n1349 = local read "Password"() -> (w2356:string)
                n1350 = String To Byte Array(string=w2356) -> (unsigned byte array=w2359:u8[])
                n1351 = String To Byte Array(string="@143$\n") -> (unsigned byte array=w2345:u8[])
                n1352 = Array Size(array=w2359) -> (size(s)=w2354:i32)
                n1353 = Array Size(array=w2345) -> (size(s)=w2350:i32)
                n1354 = for {
                  N: w2354 -> [_]
                  tunnel: w2359 -> [w2393]
                  tunnel: [w2391] -> w2360 mode=indexing
                  tunnel: w2354 -> [w2388]
                  i -> [w2389]
                  n1355 = Decrement(x=w2388) -> (x-1=w2387:i32)
                  n1356 = Index Array(array=w2393, index=w2389) -> (element=w2392:u8)
                  n1357 = Equal?(x=w2389, y=w2387) -> (x = y?=w2386:bool)
                  n1358 = Number To Decimal String(number=w2392) -> (decimal integer string=w2390:string)  [unwired: 1 in]
                  n1359 = Select(t="", s=w2386, f="\r") -> (s? t:f=w2383:string)
                  n1360 = Concatenate Strings(w2390, w2383) -> (w2391:string)
                }
                n1361 = for {
                  N: w2350 -> [_]
                  tunnel: w2345 -> [w2404]
                  tunnel: [w2402] -> w2348 mode=indexing
                  tunnel: w2350 -> [w2399]
                  i -> [w2400]
                  n1362 = Decrement(x=w2399) -> (x-1=w2398:i32)
                  n1363 = Index Array(array=w2404, index=w2400) -> (element=w2403:u8)
                  n1364 = Equal?(x=w2400, y=w2398) -> (x = y?=w2397:bool)
                  n1365 = Number To Decimal String(number=w2403) -> (decimal integer string=w2401:string)  [unwired: 1 in]
                  n1366 = Select(t="", s=w2397, f="\r") -> (s? t:f=w2394:string)
                  n1367 = Concatenate Strings(w2401, w2394) -> (w2402:string)
                }
                n1368 = local read "file path"() -> (w2344:path)
                n1369 = call <vilib>:"Read Characters From File.vi"("file path (dialog if empty)"=w2344) -> ("character string"=w2358:string)  [unwired: 5 in, 3 out]
                "string" <- w2358
                n1370 = flat-sequence {
                  tunnel: [w2361] -> w2355
                  frame #0 {
                    w2361 = ""
                    n1371 = local write "Password"(w2361) -> ()
                  }
                }
                n1372 = Concatenate Strings(w2348) -> (w2349:string)
                n1373 = Concatenate Strings(w2358) -> (w2357:string)
                n1374 = Concatenate Strings(w2360) -> (w2352:string)
                n1375 = Equal?(x=w2352, y=w2357) -> (x = y?=w2347:bool)
                n1376 = Equal?(x=w2352, y=w2349) -> (x = y?=w2353:bool)
                n1377 = Or(x=w2347, y=w2353) -> (x .or. y?=w2346:bool)
                "x = y?" <- w2346
                n1378 = case shown="True" w2346 {
                  selector: w2346 -> [w2363 _]
                  tunnel: w2355 -> [_ _]
                  frame False {
                    n1379 = And(x=w2363, y=TRUE ("Visible")) -> (x .and. y?=w2364:bool)
                    n1380 = property on="message" class="Str"("Visible"=w2364) -> ()  [unwired: 2 in, 2 out]
                  }
                  frame True {
                    n1381 = control-ref of="This VI"() -> (w2375:refnum<vi>)
                    n1382 = property class="VI"(reference=w2375) -> (reference out=w2366:refnum<vi>, error out=w2370:errorcluster, "Panel"=w2374:refnum<vi>)  [unwired: 1 in]
                    n1383 = property on="message" class="Str"("Visible"=FALSE) -> ()  [unwired: 2 in, 2 out]
                    n1384 = property class="Pnl"(reference=w2374, error in=w2370) -> (reference out=w2368:refnum<vi>, error out=w2371:errorcluster, "Panes[]"=w2373:refnum<vi>[])
                    n1385 = for {
                      tunnel: w2373 -> [w2382] mode=indexing
                      tunnel: T17."Always On" ("Horizontal Scrollbar Visibility") -> [w2381]
                      tunnel: w2371 -> [w2378]
                      tunnel: [w2377] -> w2369
                      n1386 = property class="Pane"(reference=w2382, error in=w2378, "HorizScrollbarVisibility"=w2381) -> (reference out=w2379:refnum<vi>, error out=w2380:errorcluster)
                      n1387 = Close Reference(reference=w2379, error in (no error)=w2380) -> (error out=w2377:errorcluster)
                    }
                    n1388 = Close Reference(reference=w2368, error in (no error)=w2369) -> (error out=w2367:errorcluster)
                    n1389 = Close Reference(reference=w2366, error in (no error)=w2367) -> (error out=→"error out 6":errorcluster)
                  }
                }
              }
            }
          }
        }
        n1390 = local read "x = y?"() -> (w2203:bool)
        n1391 = local read "HUMIDITY: 2"() -> (w2205:dbl)
        n1392 = local read "HUMIDITY:"() -> (w2204:dbl)
        n1393 = property on="Port 2 Error" class="Clust (strict)"("Visible"="EDIT") -> ()  [unwired: 2 in, 2 out]
        n1394 = property on="Port 1 Error" class="Clust (strict)"("Visible"="EDIT") -> ()  [unwired: 2 in, 2 out]
        n1395 = case shown="True" "SrvM CP 2" {
          frame False {
          }
          frame True {
            n1396 = local write "SrvM CP 2"(FALSE ("SrvM CP 2")) -> ()
            n1397 = local read "HUMIDITY: 2"() -> (w2244:dbl)
            n1398 = local read "TEMP INTERCEPT: 2"() -> (w2243:dbl)
            n1399 = local read "DISPLACEMENT : 4"() -> (w2247:dbl)
            n1400 = local read "TEMPERATURE : 2"() -> (w2246:dbl)
            n1401 = local read "STROKE GAIN : 2"() -> (w2248:dbl)
            n1402 = local read "FRIC. FORCE : 2"() -> (w2249:dbl)
            n1403 = local read "AIR TEMP INTERCEPT: 2"() -> (w2242:dbl)
            n1404 = local read "AIR TEMPERATURE : 2"() -> (w2245:dbl)
            n1405 = local write "HUMIDITY:"(w2244) -> ()
            n1406 = local write "AIR TEMP INTERCEPT:"(w2243) -> ()
            n1407 = local write "TEMPERATURE :"(w2246) -> ()
            n1408 = local write "FRIC. FORCE :"(w2249) -> ()
            n1409 = local write "STROKE GAIN :"(w2248) -> ()
            n1410 = local write "DISPLACEMENT :"(w2247) -> ()
            n1411 = local write "AIR TEMPERATURE :"(w2245) -> ()
            n1412 = local write "TEMP INTERCEPT:"(w2242) -> ()
          }
        }
        n1413 = Or(x="SAVE", y=w2197) -> (x .or. y?=w2198:bool)
        n1414 = And(x="EDIT", y=w2203) -> (x .and. y?=w2201:bool)
        n1415 = local read "DISPLACEMENT : 4"() -> (w2214:dbl)
        n1416 = local read "TEMPERATURE : 2"() -> (w2212:dbl)
        n1417 = local read "STROKE GAIN : 2"() -> (w2218:dbl)
        n1418 = local read "DISPLACEMENT :"() -> (w2213:dbl)
        n1419 = local read "FRIC. FORCE : 2"() -> (w2221:dbl)
        n1420 = local read "TEMPERATURE :"() -> (w2210:dbl)
        n1421 = local read "STROKE GAIN :"() -> (w2217:dbl)
        n1422 = local read "FRIC. FORCE :"() -> (w2220:dbl)
        n1423 = case shown="True" w2201 {
          tunnel: [u8 2 ("Disabled") u8 0 ("Disabled")] -> w2200
          tunnel: [w2566 TRUE ("Visible")] -> w2199
          frame False {
            w2566 = FALSE ("Visible")
            n1424 = local write "EDIT 2"(w2566) -> ()
          }
          frame True {
          }
        }
        n1425 = case shown="True" w2198 {
          frame False {
          }
          frame True {
            n1426 = stacked-sequence {
              seq-local: [w2413 _ _] -> [_ w2560 _]
              frame #0 {
                (unwired) i16 5 ("precision (6)")
                # "[CH1]    - FF\n[CH2]   - TEMPERATURE\n[CH3]    - Humidity\n[CH4]    - AIR TEMP\n[CH5]\\- Visa Uno\n[CH6] \\- Visa Due\n[CH7]  \\- file path\n[CH8]   - Displacement Gain\n[CHA]   - Stroke Gain\n[CHB]   - Stroke PID Gain\n[CHC]   -Language Selection\n[CHD]   -Power +\n[CHE]   -Power_\n[CHF]   -Heater\n[CHG]   -Humidity Wet\n[CHH]   -Humidity Dry\n[CHI]   -Integral Time"
                n1427 = local read "Language Selection"() -> (w2461:enum16{"English", "Russian"})
                n1428 = local read "CH-HUMIDITY WET"() -> (w2419:u16)
                n1429 = local read "CH-HUMIDITY DRY"() -> (w2416:u16)
                n1430 = local read "STROKE GAIN :"() -> (w2405:dbl)
                n1431 = local read "CH-POWER +"() -> (w2428:u16)
                n1432 = local read "CH-POWER -"() -> (w2425:u16)
                n1433 = local read "CH-HEATER"() -> (w2422:u16)
                n1434 = local read "AIR TEMPERATURE :"() -> (w2408:dbl)
                n1435 = local read "DISPLACEMENT :"() -> (w2406:dbl)
                n1436 = local read "TEMPERATURE :"() -> (w2409:dbl)
                n1437 = local read "FRIC. FORCE :"() -> (w2410:dbl)
                n1438 = local read "HUMIDITY:"() -> (w2407:dbl)
                n1439 = Path To String(path="File Path") -> (string=w2477:string)
                n1440 = Number To Fractional String(number=w2405, width (-)=i16 10 ("precision (6)"), precision (6)=i16 5) -> (F-format string=w2468:string)  [unwired: 1 in]
                n1441 = Number To Fractional String(number=w2461, width (-)=i16 10 ("precision (6)"), precision (6)=i16 5) -> (F-format string=w2457:string)  [unwired: 1 in]
                n1442 = Number To Fractional String(number=w2428, width (-)=i16 10 ("precision (6)"), precision (6)=i16 5) -> (F-format string=w2451:string)  [unwired: 1 in]
                n1443 = Number To Fractional String(number=w2425, width (-)=i16 10 ("precision (6)"), precision (6)=i16 5) -> (F-format string=w2448:string)  [unwired: 1 in]
                n1444 = Number To Fractional String(number=w2422, width (-)=i16 10 ("precision (6)"), precision (6)=i16 5) -> (F-format string=w2443:string)  [unwired: 1 in]
                n1445 = Number To Fractional String(number=w2419, width (-)=i16 10 ("precision (6)"), precision (6)=i16 5) -> (F-format string=w2440:string)  [unwired: 1 in]
                n1446 = Number To Fractional String(number=w2416, width (-)=i16 10 ("precision (6)"), precision (6)=i16 5) -> (F-format string=w2435:string)  [unwired: 1 in]
                n1447 = local read "Com Port 1"() -> (w2412:refnum<visa-resource-name>)
                n1448 = local read "Com Port 2"() -> (w2411:refnum<visa-resource-name>)
                n1449 = Concatenate Strings(w2477, "\\" ("string")) -> (w2476:string)
                n1450 = Number To Fractional String(number=w2410, width (-)=i16 10 ("precision (6)"), precision (6)=i16 5) -> (F-format string=w2509:string)  [unwired: 1 in]
                n1451 = Number To Fractional String(number=w2409, width (-)=i16 10 ("precision (6)"), precision (6)=i16 5) -> (F-format string=w2508:string)  [unwired: 1 in]
                n1452 = Number To Fractional String(number=w2407, width (-)=i16 10 ("precision (6)"), precision (6)=i16 5) -> (F-format string=w2502:string)  [unwired: 1 in]
                n1453 = Number To Fractional String(number=w2408, width (-)=i16 10 ("precision (6)"), precision (6)=i16 5) -> (F-format string=w2496:string)  [unwired: 1 in]
                n1454 = Number To Fractional String(number=w2406, width (-)=i16 10 ("precision (6)"), precision (6)=i16 5) -> (F-format string=w2469:string)  [unwired: 1 in]
                n1455 = Concatenate Strings("[CHA]" ("string"), w2468, "- Stroke Gain" ("string"), "\r") -> (w2462:string)
                n1456 = Concatenate Strings("[CHC]" ("string"), w2457, "-Language Selection" ("string"), "\r") -> (w2454:string)
                n1457 = Concatenate Strings("[CHD]" ("string"), w2451, "-Power +" ("string"), "\r") -> (w2433:string)
                n1458 = Concatenate Strings("[CHG]" ("string"), w2440, "-Humidity Wet" ("string"), "\r") -> (w2430:string)
                n1459 = Concatenate Strings("[CHH]" ("string"), w2435, "-Humidity Dry" ("string"), "\r") -> (w2429:string)
                n1460 = Concatenate Strings("[CH1]" ("string"), w2509, " - FF" ("string"), "\r") -> (w2507:string)
                n1461 = Concatenate Strings("[CH2]" ("string"), w2508, " - TEMPERATURE" ("string"), "\r") -> (w2506:string)
                n1462 = Concatenate Strings("[CH3]" ("string"), w2502, " - Humidity" ("string"), "\r") -> (w2499:string)
                n1463 = Concatenate Strings("[CH4]" ("string"), w2496, " - AIR TEMP" ("string"), "\r") -> (w2492:string)
                n1464 = Concatenate Strings("[CH5]" ("string"), w2412, "- Visa Uno" ("string"), "\r") -> (w2485:string)
                n1465 = Concatenate Strings("[CH6]" ("string"), w2411, "- Visa Due" ("string"), "\r") -> (w2480:string)
                n1466 = Concatenate Strings("[CH7]" ("string"), w2476, "- file path" ("string"), "\r") -> (w2479:string)
                n1467 = Concatenate Strings("[CH8]" ("string"), w2469, "- Displacement Gain" ("string"), "\r") -> (w2472:string)
                n1468 = Concatenate Strings("[CHE]" ("string"), w2448, "-Power_" ("string"), "\r") -> (w2432:string)
                n1469 = Concatenate Strings("[CHF]" ("string"), w2443, "-Heater" ("string"), "\r") -> (w2431:string)
                n1470 = Concatenate Strings(w2507, w2506, w2499, w2492, w2485, w2480, w2479, w2472, w2462, w2454, w2433, w2432, w2431, w2430, w2429) -> (w2413:string)
                "gain" <- w2413
              }
              frame #1 {
                n1471 = local read "Camera Port :"() -> (w2521:string)
                n1472 = local read "C3 :"() -> (w2529:refnum<visa-resource-name>)
                n1473 = local read "TEMP INTERCEPT:"() -> (w2530:dbl)
                n1474 = local read "AIR TEMP INTERCEPT:"() -> (w2531:dbl)
                n1475 = Concatenate Strings("[CH8]" ("string"), w2521, "- Visa Camera" ("string"), "\r") -> (w2520:string)
                n1476 = Concatenate Strings("[CH7]" ("string"), w2529, "- Visa Humidity" ("string"), "\r") -> (w2525:string)
                n1477 = Number To Fractional String(number=w2530, width (-)=i16 10 ("precision (6)"), precision (6)=i16 5) -> (F-format string=w2548:string)  [unwired: 1 in]
                n1478 = local read "Com Port 3"() -> (w2532:refnum<visa-resource-name>)
                n1479 = Number To Fractional String(number=w2531, width (-)=i16 10 ("precision (6)"), precision (6)=i16 5) -> (F-format string=w2555:string)  [unwired: 1 in]
                n1480 = Concatenate Strings("[CHK]" ("string"), w2548, "-TEMP INTERCEPT" ("string"), "\r") -> (w2544:string)
                n1481 = Concatenate Strings("[SNO]" ("string"), "S.NO", "-" ("string"), "\r") -> (w2540:string)
                n1482 = Concatenate Strings("[CHJ]" ("string"), w2555, "-AIR TEMP INTERCEPT" ("string"), "\r") -> (w2545:string)
                n1483 = Concatenate Strings("[CHL]" ("string"), w2532, "- Visa humid" ("string"), "\r") -> (w2535:string)
                n1484 = String To Path(string="C:\\LAB-IQ\\calibrate WO 2465.dcf") -> (path=w2533:path)
                n1485 = Concatenate Strings(w2560, w2545, w2544, w2540, w2535, w2525, w2520) -> (w2559:string)
                n1486 = call <vilib>:"Write Characters To File.vi"("append to file? (new file:F)"=FALSE, "character string"=w2559, "file path (dialog if empty)"=w2533) -> ()  [unwired: 2 in, 1 out]
              }
              frame #2 {
                n1487 = local write "Lan flag"(0.0 ("Lan flag")) -> ()
                n1488 = local write "conststatus"(0.0 ("rpm value : 2")) -> ()
                n1489 = local write "SAVE"(FALSE ("OK Button 14")) -> ()
                n1490 = local write "Re-Initialise"(TRUE ("Re-Initialise")) -> ()
                n1491 = local write "SAVE 2"(FALSE ("SAVE 2")) -> ()
              }
            }
          }
        }
        n1492 = Subtract(x=w2205, y=w2204) -> (x-y=w2206:dbl)
        n1493 = local read "AIR TEMPERATURE : 2"() -> (w2209:dbl)
        n1494 = local read "AIR TEMPERATURE :"() -> (w2208:dbl)
        n1495 = Divide(x=w2206, y=w2204) -> (x/y=w2228:dbl)
        n1496 = Subtract(x=w2221, y=w2220) -> (x-y=w2219:dbl)
        n1497 = Subtract(x=w2212, y=w2210) -> (x-y=w2211:dbl)
        n1498 = Subtract(x=w2218, y=w2217) -> (x-y=w2216:dbl)
        n1499 = Subtract(x=w2214, y=w2213) -> (x-y=w2215:dbl)
        n1500 = Subtract(x=w2209, y=w2208) -> (x-y=w2207:dbl)
        n1501 = Divide(x=w2219, y=w2220) -> (x/y=w2239:dbl)
        n1502 = Divide(x=w2211, y=w2210) -> (x/y=w2232:dbl)
        n1503 = Divide(x=w2216, y=w2217) -> (x/y=w2236:dbl)
        n1504 = Divide(x=w2215, y=w2213) -> (x/y=w2235:dbl)
        n1505 = Multiply(x=w2228, y=100.0) -> (x*y=→"HUMIDITY  Calibration Error":dbl)
        n1506 = Divide(x=w2207, y=w2208) -> (x/y=w2231:dbl)
        n1507 = Multiply(x=w2239, y=100.0) -> (x*y=→"FRIC. FORCE Calibration Error":dbl)
        n1508 = Multiply(x=w2232, y=100.0) -> (x*y=→"TEMPERATURE  Calibration Error":dbl)
        n1509 = Multiply(x=w2236, y=100.0) -> (x*y=→"STROKE Calibration Error":dbl)
        n1510 = Multiply(x=w2235, y=100.0) -> (x*y=→"DISPLACEMENT  Calibration Error":dbl)
        n1511 = property on="EDIT 2" class="Bool (strict)"("Visible"=w2199) -> ()  [unwired: 2 in, 2 out]
        n1512 = property on="SAVE" class="Bool (strict)"("Visible"=w2199) -> ()  [unwired: 2 in, 2 out]
        n1513 = property on="SrvM CP" class="Bool (strict)"("Disabled"=w2200) -> ()  [unwired: 2 in, 2 out]
        n1514 = property on="visa due" class="CmbBox"("Disabled"=w2200) -> ()  [unwired: 2 in, 2 out]
        n1515 = property on="File Path" class="Path"("Disabled"=w2200) -> ()  [unwired: 2 in, 2 out]
        n1516 = Multiply(x=w2231, y=100.0) -> (x*y=→"AIR TEMPERATURE  Calibration Error":dbl)
        n1517 = property on="Tab Control" class="TabCtl (strict)"("Visible"=w2199) -> ()  [unwired: 2 in, 2 out]
        n1518 = property on="Language Selection" class="Enum (strict)"("Visible"=w2199) -> ()  [unwired: 2 in, 2 out]
        n1519 = property on="Tab Control 7" class="TabCtl (strict)"("Disabled"=w2200) -> ()  [unwired: 2 in, 2 out]
        n1520 = property on="AIR TEMP INTERCEPT:" class="DigNum (strict)"("Disabled"=w2200) -> ()  [unwired: 2 in, 2 out]
        n1521 = property on="CH-POWER -" class="DigNum (strict)"("Disabled"=w2200) -> ()  [unwired: 2 in, 2 out]
        n1522 = property on="CH-POWER +" class="DigNum (strict)"("Disabled"=w2200) -> ()  [unwired: 2 in, 2 out]
        n1523 = property on="AIR TEMPERATURE :" class="DigNum (strict)"("Disabled"=w2200) -> ()  [unwired: 2 in, 2 out]
        n1524 = property on="STROKE GAIN :" class="DigNum (strict)"("Disabled"=w2200) -> ()  [unwired: 2 in, 2 out]
        n1525 = property on="SPEED OUT:" class="DigNum (strict)"("Disabled"=w2200) -> ()  [unwired: 2 in, 2 out]
        n1526 = property on="CH-HUMIDITY DRY" class="DigNum (strict)"("Disabled"=w2200) -> ()  [unwired: 2 in, 2 out]
        n1527 = property on="HUMIDITY:" class="DigNum (strict)"("Disabled"=w2200) -> ()  [unwired: 2 in, 2 out]
        n1528 = property on="CH-HUMIDITY WET" class="DigNum (strict)"("Disabled"=w2200) -> ()  [unwired: 2 in, 2 out]
        n1529 = property on="TEMPERATURE :" class="DigNum (strict)"("Disabled"=w2200) -> ()  [unwired: 2 in, 2 out]
        n1530 = property on="DISPLACEMENT :" class="DigNum (strict)"("Disabled"=w2200) -> ()  [unwired: 2 in, 2 out]
        n1531 = property on="CH-HEATER" class="DigNum (strict)"("Disabled"=w2200) -> ()  [unwired: 2 in, 2 out]
        n1532 = property on="TEMP INTERCEPT:" class="DigNum (strict)"("Disabled"=w2200) -> ()  [unwired: 2 in, 2 out]
        n1533 = property on="FRIC. FORCE :" class="DigNum (strict)"("Disabled"=w2200) -> ()  [unwired: 2 in, 2 out]
      }
    }
    n1534 = local read "RUN"() -> (w1593:bool)
    n1535 = local read "RUN"() -> (w1591:bool)
    n1536 = disable-structure shown="Disabled" {
      disable-tunnel: [w1608 _] -> w1573
      disable-tunnel: [w1607 _] -> w1571
      frame Disabled {
        n1537 = local read "Temperature before test"() -> (w1601:dbl)
        n1538 = local read "Temperature after test"() -> (w1614:dbl)
        n1539 = case shown="True" "Save Results" {
          frame False {
          }
          frame True {
            w1630 = "\r"
            n1540 = local write "Save Results"(FALSE ("OK Button 5")) -> ()
            n1541 = local read "Temperature before test"() -> (w1668:dbl)
            n1542 = local read "Temperature after test"() -> (w1670:dbl)
            n1543 = local read "Humidity before test"() -> (w1667:dbl)
            n1544 = local read "Humidity after test"() -> (w1669:dbl)
            n1545 = local read "WS1.4"() -> (w1674:dbl)
            n1546 = local read "AVP"() -> (w1672:dbl)
            n1547 = Number To Fractional String(number=w1674, width (-)=i16 6, precision (6)=i16 1) -> (F-format string=w1634:string)  [unwired: 1 in]
            n1548 = local read "MWSD"() -> (w1671:dbl)
            n1549 = local read "String"() -> (w1663:string)
            n1550 = local read "FILE"() -> (w1666:string)
            n1551 = local read "HCF"() -> (w1673:dbl)
            n1552 = Number To Fractional String(number=w1667, width (-)=i16 6, precision (6)=i16 1) -> (F-format string=w1659:string)  [unwired: 1 in]
            n1553 = Number To Fractional String(number=w1668, width (-)=i16 6, precision (6)=i16 1) -> (F-format string=w1656:string)  [unwired: 1 in]
            n1554 = Number To Fractional String(number=w1669, width (-)=i16 6, precision (6)=i16 1) -> (F-format string=w1652:string)  [unwired: 1 in]
            n1555 = Number To Fractional String(number=w1670, width (-)=i16 6, precision (6)=i16 1) -> (F-format string=w1648:string)  [unwired: 1 in]
            n1556 = Number To Fractional String(number=w1672, width (-)=i16 6, precision (6)=i16 3) -> (F-format string=w1641:string)  [unwired: 1 in]
            n1557 = Concatenate Strings(w1663, w1666) -> (w1685:string)
            n1558 = Number To Fractional String(number=w1671, width (-)=i16 6, precision (6)=i16 1) -> (F-format string=w1645:string)  [unwired: 1 in]
            n1559 = Number To Fractional String(number=w1673, width (-)=i16 6, precision (6)=i16 2) -> (F-format string=w1639:string)  [unwired: 1 in]
            n1560 = Concatenate Strings("(" ("string"), w1634, ")Microns" ("string")) -> (w1633:string)
            n1561 = local read "REMARKS"() -> (w1665:string)
            "REMARKS 2" <- w1665
            n1562 = Concatenate Strings("(" ("string"), w1659, " ) % RH," ("string")) -> (w1660:string)
            n1563 = Concatenate Strings(w1639, ")" ("string")) -> (w1637:string)
            n1564 = Concatenate Strings("(" ("string"), w1656, ")  Deg C ," ("string")) -> (w1655:string)
